vi "Configure Multi Eval Meas Limit IQ Offset.vi"(5 "Offset 1 (-20.0)":dbl=-20.0 format="%^.3e", 6 "Offset 0 (-25.0)":dbl=-25.0 format="%^.3e", 7 "Enable (On)":bool=TRUE, 8 "error in (no error)":errorcluster, 9 "Modulation (Pi/2-BPSK)":i32(ring) items=["Pi/2-BPSK", "QPSK", "16-QAM", "64-QAM", "256-QAM"], 10 "Instance (1)":T1=1, 11 "VISA resource name":refnum<visa-resource-name>) -> (0 "error out":errorcluster, 3 "VISA resource name out":refnum<visa-resource-name>)   [LabVIEW 2020, in "Rohde&Schwarz CMXP NR FR2 Measurement.lvlib"]
doc: "Defines upper limits for the I/Q origin offset. Two different I/Q origin offset limits can be set for two TX power ranges.\n\nAttributes:\nRSCMXPNRFR2M_ATTR_MULTI_EVAL_MEASUREMENT_LIMIT_PHBPSK_IQ_OFFSET\nRSCMXPNRFR2M_ATTR_MULTI_EVAL_MEASUREMENT_LIMIT_QPSK_IQ_OFFSET\nRSCMXPNRFR2M_ATTR_MULTI_EVAL_MEASUREMENT_LIMIT_QAM16_IQ_OFFSET\nRSCMXPNRFR2M_ATTR_MULTI_EVAL_MEASUREMENT_LIMIT_QAM64_IQ_OFFSET\nRSCMXPNRFR2M_ATTR_MULTI_EVAL_MEASUREMENT_LIMIT_QAM256_IQ_OFFSET\n\nRemote-control commands:\nCONFigure:NRMMw:MEAS<i>:MEValuation:LIMit:PHBPsk:IQOFfset\nCONFigure:NRMMw:MEAS<i>:MEValuation:LIMit:QPSK:IQOFfset\nCONFigure:NRMMw:MEAS<i>:MEValuation:LIMit:QAM<order>:IQOFfset"
uses:
  <instrlib>/Rohde&Schwarz CMXP NR FR2 Measurement/Rohde&Schwarz CMXP NR FR2 Measurement.lvlib
  <instrlib>/Rohde&Schwarz CMXP NR FR2 Measurement/Private/_Instance.ctl
  <instrlib>/Rohde&Schwarz CMXP NR FR2 Measurement/Private/rsidr_core.llb/rsidr_core.lvlib
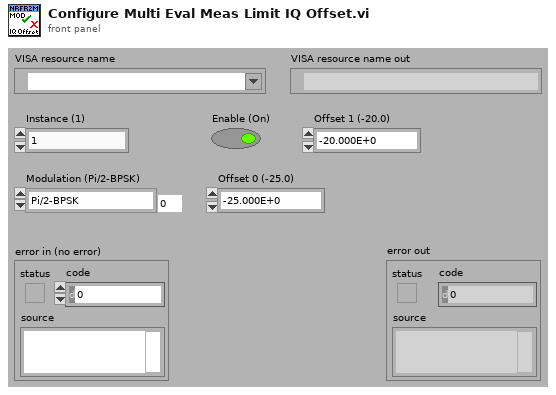
[diagram p1: front panel]
types:
  T1 = typedef "Rohde&Schwarz CMXP NR FR2 Measurement.lvlib/_Instance.ctl" = i32
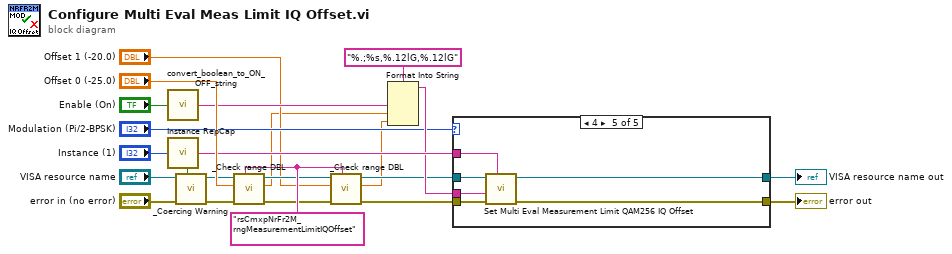
[diagram p0: block diagram]
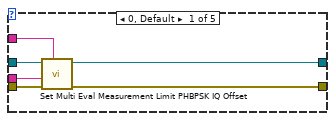
[diagram p2: hidden frame]
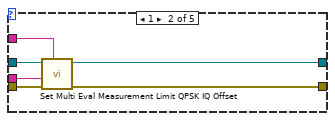
[diagram p3: hidden frame]
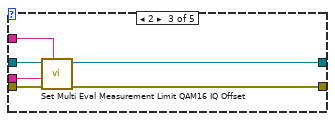
[diagram p4: hidden frame]
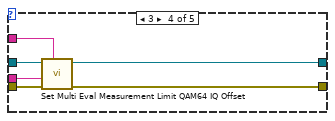
[diagram p5: hidden frame]
diagram:
  w20 = "rsCmxpNrFr2M_rngMeasurementLimitIQOffset"
  n1 = call <instrlib>:"convert_boolean_to_ON_OFF_string.vi"("boolean value in"="Enable (On)") -> ("string value out"=w11:string)  [unwired: 4 in]
  n2 = call <instrlib>:"Instance RepCap.vi"("Instance In"="Instance (1)") -> ("In Range?"=w21:bool, "RepCap Identifier Out"=w14:string)  [unwired: 1 in]
  n3 = call <instrlib>:"_Coercing Warning.vi"("In Range?"=w21, "error in (no error)"="error in (no error)", "VISA resource name"="VISA resource name") -> ("error out"=w17:errorcluster, "VISA resource name out"=w18:refnum<visa-resource-name>)  [unwired: 7 in]
  n4 = call <instrlib>:"_Check range DBL.vi"("Range Table Identifier"=w20, "error in (no error)"=w17, "DBL Value In"="Offset 0 (-25.0)", "VISA resource name"=w18) -> ("error out"=w15:errorcluster, "DBL Value Out"=w3:dbl, "VISA resource name out"=w16:refnum<visa-resource-name>)  [unwired: 5 in]
  n5 = call <instrlib>:"_Check range DBL.vi"("Range Table Identifier"=w20, "error in (no error)"=w15, "DBL Value In"="Offset 1 (-20.0)", "VISA resource name"=w16) -> ("error out"=w9:errorcluster, "DBL Value Out"=w2:dbl, "VISA resource name out"=w8:refnum<visa-resource-name>)  [unwired: 5 in]
  n6 = Format Into String(format string="%.;%s,%.12lG,%.12lG", w11, w3, w2) -> (resulting string=w10:string)  [unwired: 2 in, 1 out]
  n7 = case shown="4" "Modulation (Pi/2-BPSK)" {
    tunnel: w14 -> [w29 w35 w41 w47 w53]
    tunnel: w10 -> [w24 w30 w36 w42 w48]
    tunnel: w9 -> [w28 w34 w40 w46 w52]
    tunnel: w8 -> [w27 w33 w39 w45 w51]
    tunnel: [w26 w32 w38 w44 w50] -> w7
    tunnel: [w25 w31 w37 w43 w49] -> w6
    frame 0, Default {
      n8 = call "Set Multi Eval Measurement Limit PHBPSK IQ Offset"("Repeated Capabilities"=w29, "error in (no error)"=w28, "Multi Eval Measurement Limit PHBPSK IQ Offset ()"=w24, "instrument handle"=w27) -> ("error out"=w26:errorcluster, "instrument handle out"=w25:refnum<visa-resource-name>)  [unwired: 6 in]
    }
    frame 1 {
      n9 = call "Set Multi Eval Measurement Limit QPSK IQ Offset"("Repeated Capabilities"=w35, "error in (no error)"=w34, "Multi Eval Measurement Limit QPSK IQ Offset ()"=w30, "instrument handle"=w33) -> ("error out"=w32:errorcluster, "instrument handle out"=w31:refnum<visa-resource-name>)  [unwired: 6 in]
    }
    frame 2 {
      n10 = call "Set Multi Eval Measurement Limit QAM16 IQ Offset"("Repeated Capabilities"=w41, "error in (no error)"=w40, "Multi Eval Measurement Limit QAM16 IQ Offset ()"=w36, "instrument handle"=w39) -> ("error out"=w38:errorcluster, "instrument handle out"=w37:refnum<visa-resource-name>)  [unwired: 6 in]
    }
    frame 3 {
      n11 = call "Set Multi Eval Measurement Limit QAM64 IQ Offset"("Repeated Capabilities"=w47, "error in (no error)"=w46, "Multi Eval Measurement Limit QAM64 IQ Offset ()"=w42, "instrument handle"=w45) -> ("error out"=w44:errorcluster, "instrument handle out"=w43:refnum<visa-resource-name>)  [unwired: 6 in]
    }
    frame 4 {
      n12 = call "Set Multi Eval Measurement Limit QAM256 IQ Offset"("Repeated Capabilities"=w53, "error in (no error)"=w52, "Multi Eval Measurement Limit QAM256 IQ Offset ()"=w48, "instrument handle"=w51) -> ("error out"=w50:errorcluster, "instrument handle out"=w49:refnum<visa-resource-name>)  [unwired: 6 in]
    }
  }
  "error out" <- w7
  "VISA resource name out" <- w6
